vi "题目三.vi"(2 "停止":bool, 3 "温度单位":bool) -> (0 "温度":string, 1 "温度计":dbl(slide) scale=0.0..260.0)   [LabVIEW 2017]
panel:
  # "℉"
  # "℃"
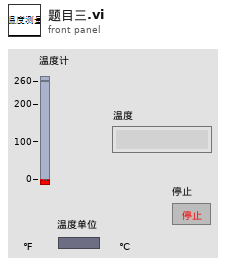
[diagram p1: front panel]
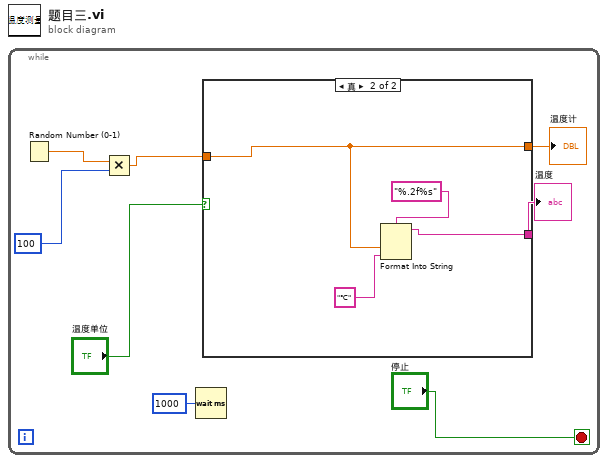
[diagram p0: block diagram]
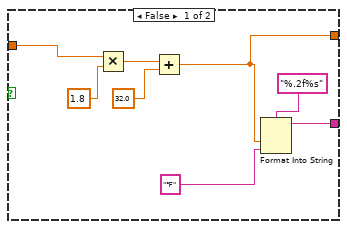
[diagram p2: hidden frame]
diagram:
  n1 = while {
    stop <- "停止" stop-if-true
    n2 = Random Number (0-1)() -> (number: 0 to 1=w3:dbl)
    n3 = Multiply(x=w3, y=100) -> (x*y=w6:dbl)
    n4 = Wait (ms)(milliseconds to wait=u32 1000 ("等待时间（毫秒）")) -> ()  [unwired: 1 out]
    n5 = case shown="真" "温度单位" {
      tunnel: w6 -> [w13 w19]
      tunnel: [w10 w19] -> w5
      tunnel: [w11 w18] -> w4
      frame False {
        n6 = Multiply(x=w13, y=1.8) -> (x*y=w15:dbl)
        n7 = Add(x=w15, y=32.0) -> (x+y=w10:dbl)
        n8 = Format Into String(format string="%.2f%s", w10, "℉") -> (resulting string=w11:string)  [unwired: 2 in, 1 out]
      }
      frame True {
        n9 = Format Into String(format string="%.2f%s", w19, "℃") -> (resulting string=w18:string)  [unwired: 2 in, 1 out]
      }
    }
    "温度" <- w4
    "温度计" <- w5
  }
